vi "uMsg_Delayed Daemon.vi"(11 "uMsg_Delayed in":refnum<class "uMsg_Delayed.lvclass">) -> ()   [LabVIEW 2023, in "uLib.lvlib" / "uMsg_Delayed.lvclass"]
uses:
  uMsg_Delayed.lvclass
  uMsg_Delayed.lvclass/uMsg_Delayed.ctl
  uMsg/uMsg.lvclass/uMsg.ctl
  uMsg/uMsg Update Timestamp.vi
  uTransport/uTransport/uTransport.lvclass
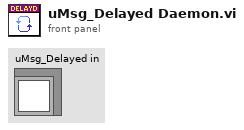
[diagram p1: front panel]
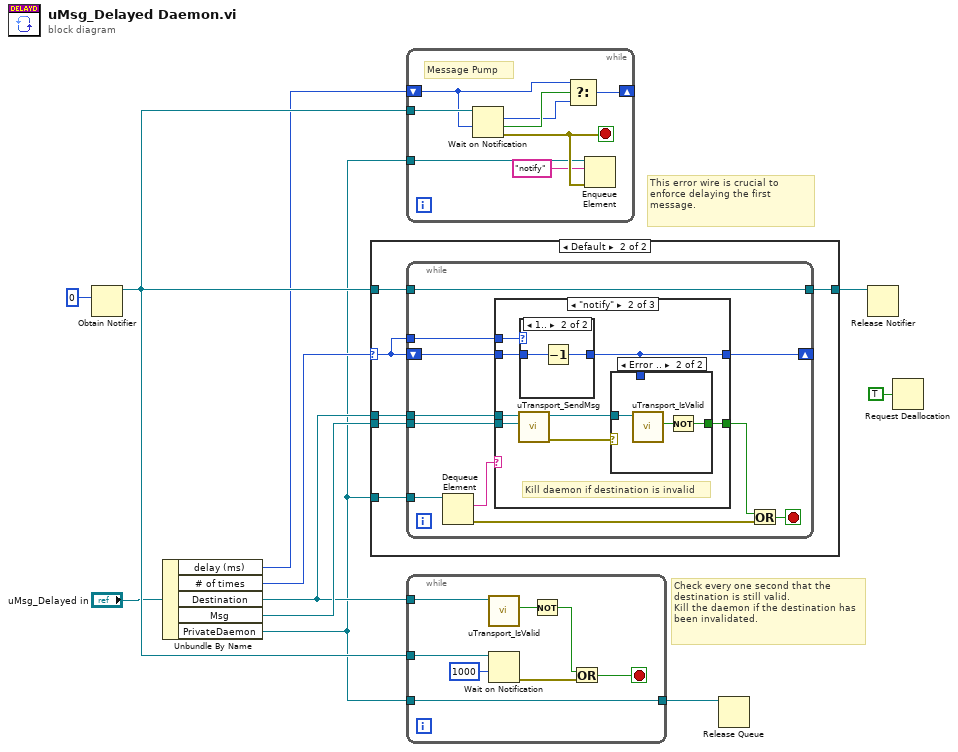
[diagram p0: block diagram]
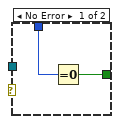
[diagram p5: hidden frame]
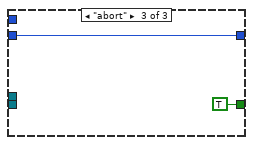
[diagram p6: hidden frame]
diagram:
  # "This error wire is crucial to enforce delaying the first message."
  # "Check every one second that the destination is still valid.\nKill the daemon if the destination has been invalidated."
  n1 = Obtain Notifier(notification data type=0) -> (notifier out=w9:refnum<notifier>)  [unwired: 3 in, 2 out]
  n2 = Unbundle By Name("uMsg_Delayed in") -> ("delay (ms)"=w6:i32, "# of times"=w5:i32, "Destination"=w3:refnum<class "uTransport.lvclass">, "Msg"=w4:refnum<class "uMsg.lvclass">, "PrivateDaemon"=w2:refnum<queue>)
  n3 = case shown="Default" w5 {
    selector: w5 -> [_ w14]
    tunnel: [w12 w18] -> w10
    tunnel: w9 -> [w12 w17]
    tunnel: w2 -> [_ w16]
    tunnel: w4 -> [_ w15]
    tunnel: w3 -> [_ w13]
    frame 0 {
    }
    frame Default {
      n4 = while {
        tunnel: w16 -> [w29]
        tunnel: w17 -> [w27]
        tunnel: [w27] -> w18
        tunnel: w15 -> [w26]
        shift-right: [w22] -> _
        shift-left: w14 -> [w25]
        tunnel: w14 -> [w23]
        tunnel: w13 -> [w24]
        stop <- w28 stop-if-true
        n5 = Dequeue Element(queue=w29) -> (element=w20:string, error out=w19:errorcluster)  [unwired: 2 in, 2 out]
        n6 = case shown="\"notify\"" w20 {
          tunnel: [_ w36 TRUE] -> w21
          tunnel: w26 -> [_ w35 _]
          tunnel: w25 -> [w30 w33 w48]
          tunnel: [w30 w31 w48] -> w22
          tunnel: w24 -> [_ w34 _]
          tunnel: w23 -> [_ w32 _]
          frame Default {
          }
          frame "notify" {
            # "Kill daemon if destination is invalid"
            n7 = call "uTransport_SendMsg.vi"("Msg"=w35, "uTransport in"=w34) -> ("error out"=w38:errorcluster, "uTransport out"=w37:refnum<class "uTransport.lvclass">)  [unwired: 8 in]
            n8 = case shown="1.." w32 {
              tunnel: [w39 w41] -> w31
              tunnel: w33 -> [w39 w40]
              frame ..0 {
              }
              frame 1.. {
                n9 = Decrement(x=w40) -> (x-1=w41:i32)
              }
            }
            n10 = case shown="Error .." w38 {
              tunnel: w37 -> [_ w46]
              tunnel: [w43 w44] -> w36
              tunnel: w31 -> [w42 _]
              frame No Error {
                n11 = Equal To 0?(x=w42) -> (x = 0?=w43:bool)
              }
              frame Error {
                n12 = call-dynamic "uTransport_IsValid.vi"("uTransport in"=w46) -> ("IsValid?"=w45:bool)  [unwired: 8 in, 2 out]
                n13 = Not(x=w45) -> (.not. x?=w44:bool)
              }
            }
          }
          frame "abort" {
          }
        }
        n14 = Or(x=w21, y=w19) -> (x .or. y?=w28:bool)
      }
    }
  }
  n15 = while {
    tunnel: w9 -> [w55]
    tunnel: w2 -> [w54]
    shift-right: [w51] -> _
    shift-left: w6 -> [w52]
    stop <- w56 stop-if-true
    # "Message Pump"
    n16 = Wait on Notification(notifier=w55, timeout in ms (-1)=w52) -> (notification=w50:i32, timed out?=w53:bool, error out=w56:errorcluster)  [unwired: 2 in, 1 out]
    n17 = Select(t=w52, s=w53, f=w50) -> (s? t:f=w51:i32)
    n18 = Enqueue Element(queue=w54, element="notify" ("CMD"), error in (no error)=w56) -> ()  [unwired: 1 in, 3 out]
  }
  n19 = while {
    tunnel: w2 -> [w64]
    tunnel: [w64] -> w11
    tunnel: w9 -> [w59]
    tunnel: w3 -> [w57]
    stop <- w62 stop-if-true
    n20 = call-dynamic "uTransport_IsValid.vi"("uTransport in"=w57) -> ("IsValid?"=w61:bool)  [unwired: 8 in, 2 out]
    n21 = Wait on Notification(notifier=w59, timeout in ms (-1)=1000) -> (error out=w63:errorcluster)  [unwired: 2 in, 3 out]
    n22 = Not(x=w61) -> (.not. x?=w60:bool)
    n23 = Or(x=w60, y=w63) -> (x .or. y?=w62:bool)
  }
  n24 = Release Queue(queue=w11) -> ()  [unwired: 2 in, 3 out]
  n25 = Release Notifier(notifier=w10) -> ()  [unwired: 2 in, 3 out]
  n26 = Request Deallocation(TRUE ("flag")) -> ()
